vi "Close Scripting References.vi"(8 "error in":errorcluster, 11 "Selection Info":T1) -> (0 "error out":errorcluster)   [LabVIEW 2020, in "ConstantErrorsMaker.lvlib"]
uses:
  ConstantErrorsMaker.lvlib
  Selection Info--cluster.ctl
  Selection Type--enum.ctl
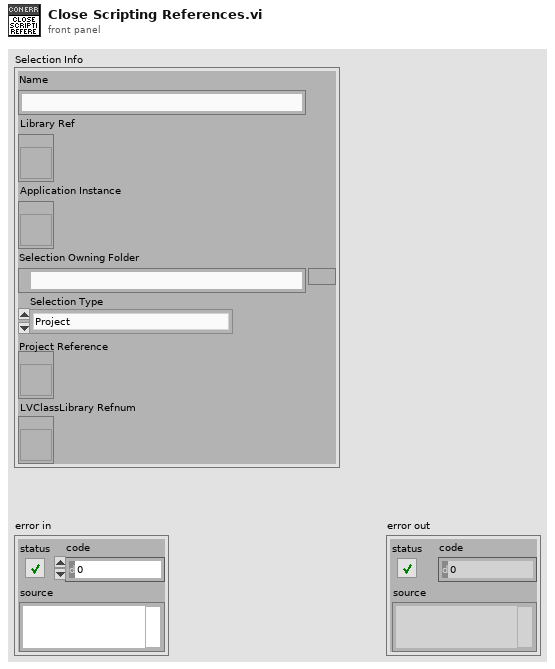
[diagram p1: front panel]
types:
  T1 = typedef "ConstantErrorsMaker.lvlib/Selection Info--cluster.ctl" = cluster{"Name":string, "Library Ref":refnum<vi>, "Application Instance":refnum<vi>, "Selection Owning Folder":path, "Selection Type":T2, "Project Reference":refnum<vi>, "LVClassLibrary Refnum":refnum<vi>}
  T2 = typedef "ConstantErrorsMaker.lvlib/Selection Type--enum.ctl" = enum16{"Project", "Library", "Class", "DQMH Module Singleton", "DQMH Module Cloneable"}
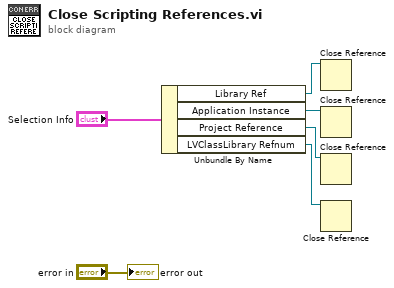
[diagram p0: block diagram]
diagram:
  n1 = Unbundle By Name("Selection Info") -> ("Library Ref"=w4:refnum<vi>, "Application Instance"=w3:refnum<vi>, "Project Reference"=w2:refnum<vi>, "LVClassLibrary Refnum"=w1:refnum<vi>)
  n2 = Close Reference(reference=w4) -> ()  [unwired: 1 in, 1 out]
  n3 = Close Reference(reference=w3) -> ()  [unwired: 1 in, 1 out]
  n4 = Close Reference(reference=w2) -> ()  [unwired: 1 in, 1 out]
  n5 = Close Reference(reference=w1) -> ()  [unwired: 1 in, 1 out]
  "error out" <- "error in"
